vi "Untitled 1.vi"() -> ()   [LabVIEW 2018]
uses:
  C:/Users/bowenm/Git/Acquisition/Instruments/ImagingPyrometer/Kineses/Thorlabs.MotionControl.Controls.dll
  Kineses/Thorlabs.MotionControl.Controls.dll
  C:/Users/bowenm/Git/Acquisition/Instruments/ImagingPyrometer/Kineses/ThorLabs.MotionControl.KCube.DCServoCLI.dll
  Kineses/ThorLabs.MotionControl.KCube.DCServoCLI.dll
  Global Variables.vi
  <vilib>/Utility/file.llb/Read Delimited Spreadsheet (string).vi
  <instrlib>/Thorlabs_FW102C/Thorlabs_FW102C.lvlib
panel:
  in  "Stop":bool
  out "NDFW102C out 2":i32
  out "tdms file out 2":refnum<k34>
  out "RFW102C out 2":i32=1
  out "TFW102C out 2":i32
  out "MotorMoving 2":bool
  out "Device 2":refnum<k24>
  in  "KCubeDCServoControl 2":refnum<k24>(container)
  out "NDFW102C out":i32
  in  "NDFW Serial Port":string="COM5"
  out "tdms file out":refnum<k34>
  out "RFW wls":string[](array[string])=["1000", "850", "800", "700", "650", "600"]
  out "TFW wls":string[](array[string])=["900", "850", "800", "750", "700", "600"]
  in  "Tab Control":enum32{"400-700nm", "700-1100nm"}(tab)
  in  "VisTFW Wavelength":u16(ring) caption="Wavelength 1" items=["600", "700"]
  in  "VisRFW Wavelength":u16(ring) caption="Wavelength 2" items=["600", "650", "700"]
  in  "NIRRFW Wavelengths":u16(ring) caption="Wavelength 2" items=["700", "800", "850", "1000"]
  in  "NIRTFW Wavelengths":u16(ring) caption="Wavelength 1" items=["700", "750", "800", "850", "900"]
  out "NDFs":dbl[](array[numeric])=[0.0, 0.2, 0.4, 0.5, 0.6, 1.0]
  in  "NeutralDensityFilter":u16(ring) items=["0", "0.2", "0.4", "0.5", "0.6", "1"]
  out "RFW102C out":i32=1
  in  "RFW Serial Port":string="COM3"
  out "error out":errorcluster
  out "TFW102C out":i32
  in  "TFW Serial Port":string="COM4"
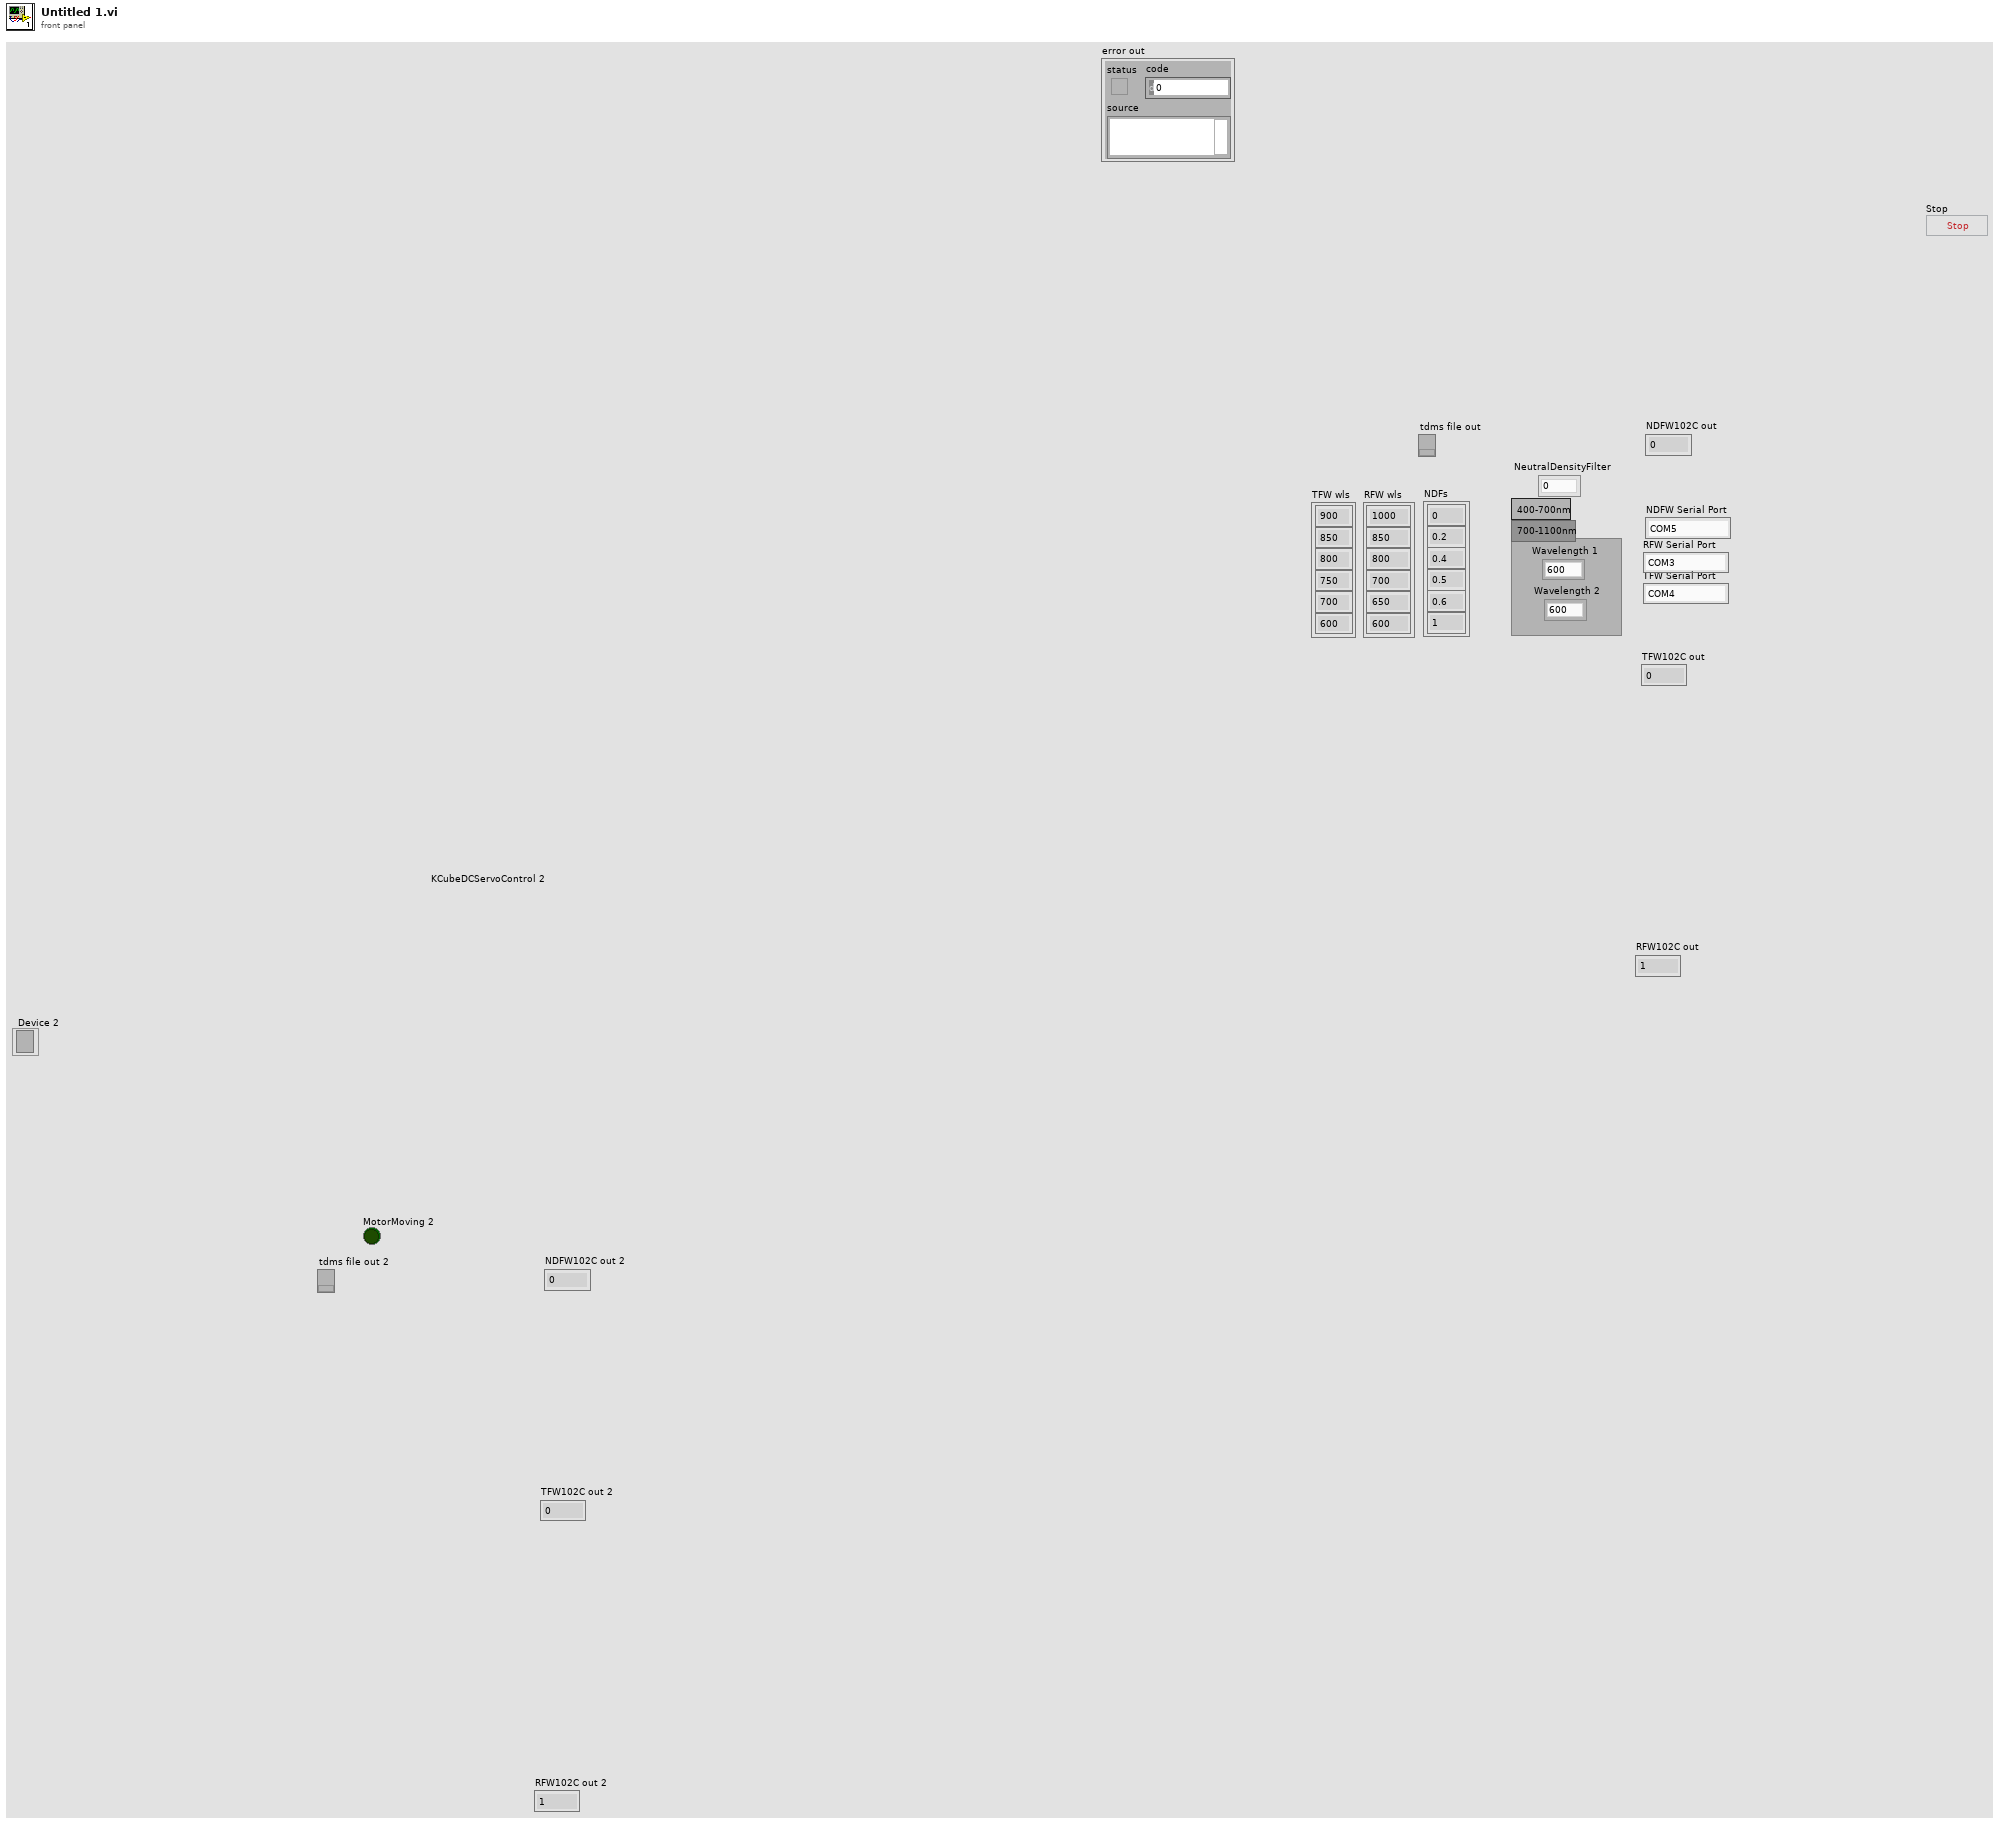
[diagram p1: front panel]
types:
  T1 = enum16{"open", "open or create", "create or replace", "create", "open (read-only)"}
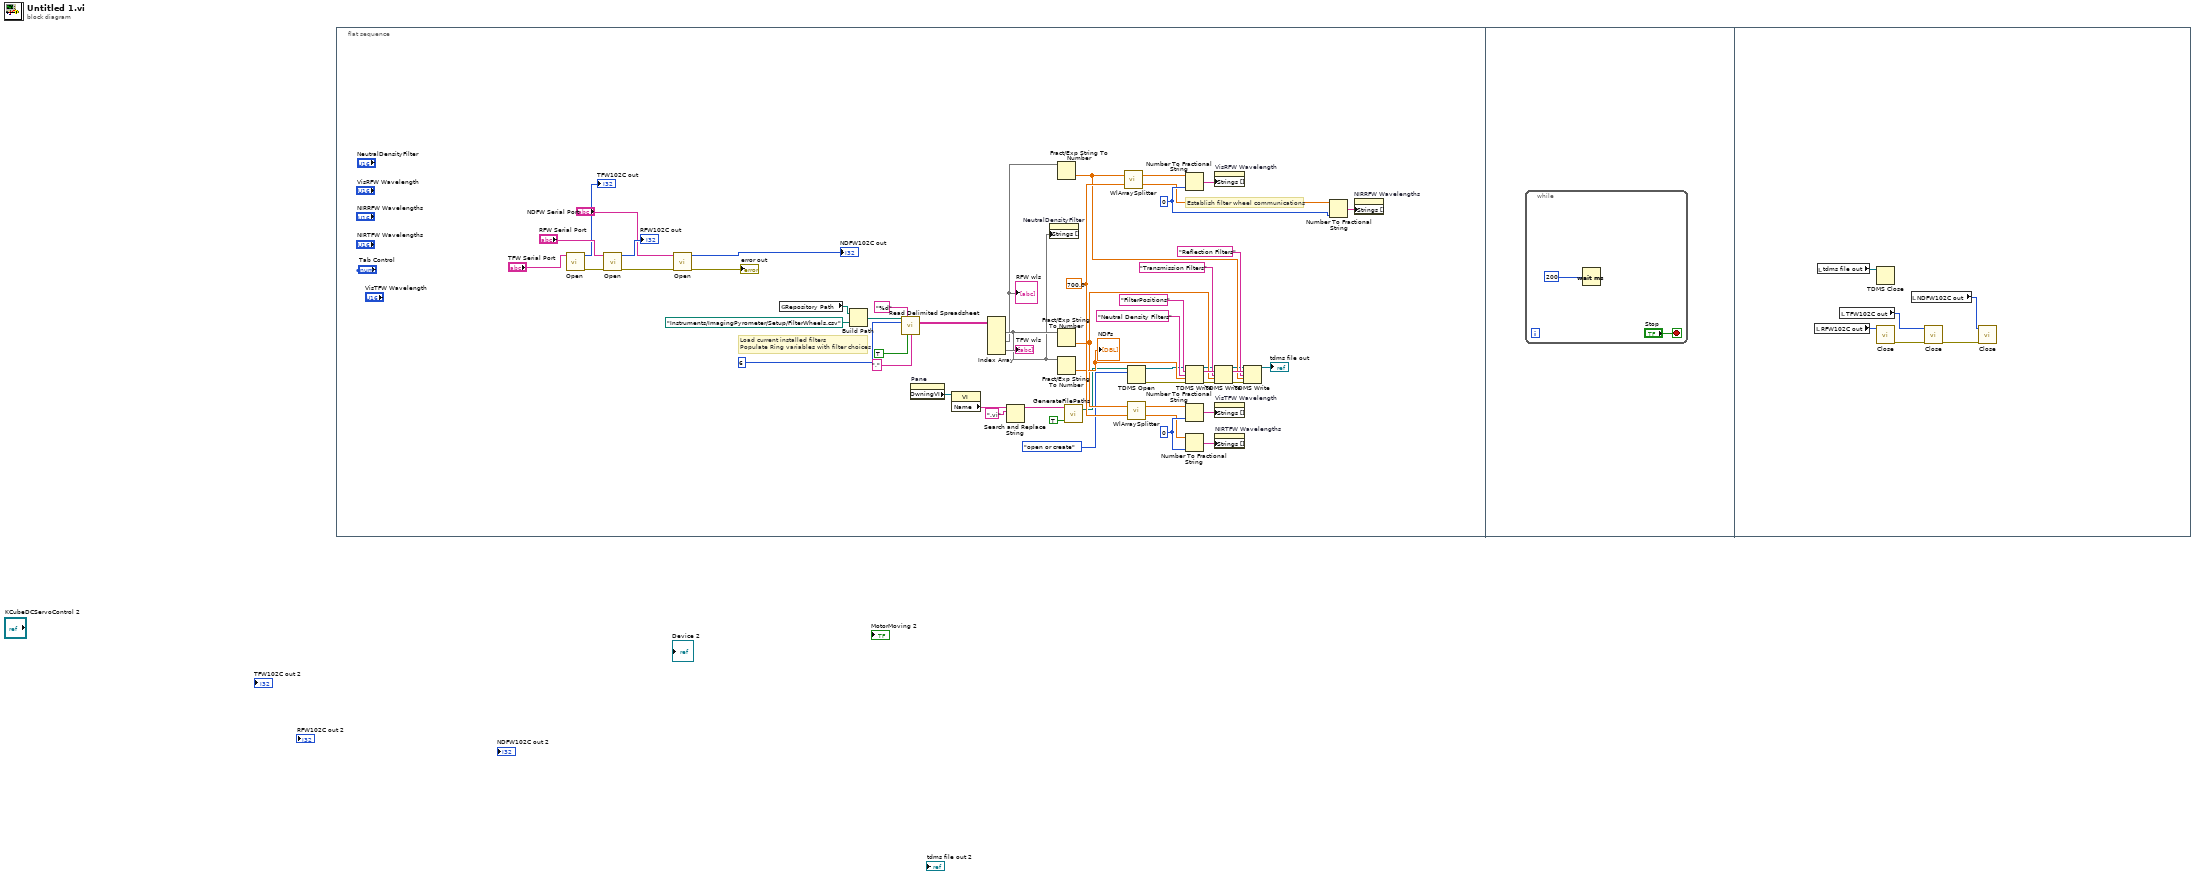
[diagram p0: block diagram]
diagram:
  n1 = flat-sequence {
    frame #0 {
      w31 = i16 0 ("precision (6)")
      w32 = 700.0 ("Cutoff Wavelength")
      w41 = i16 0 ("precision (6)")
      # "Load current installed filters\nPopulate Ring variables with filter choices"
      # "Establish filter wheel communications"
      n2 = call <instrlib>:"Open.vi"("Serial Port"="TFW Serial Port") -> ("error out"=w52:errorcluster, "FW102C out"=→"TFW102C out":i32)  [unwired: 8 in, 1 out]
      n3 = call <instrlib>:"Open.vi"("error in (no error)"=w52, "Serial Port"="RFW Serial Port") -> ("error out"=w53:errorcluster, "FW102C out"=→"RFW102C out":i32)  [unwired: 7 in, 1 out]
      n4 = call <instrlib>:"Open.vi"("error in (no error)"=w53, "Serial Port"="NDFW Serial Port") -> ("error out"=→"error out":errorcluster, "FW102C out"=→"NDFW102C out":i32)  [unwired: 7 in, 1 out]
      n5 = global read "Global Variables.vi" "Repository Path"() -> (w43:path)
      n6 = Build Path(base path=w43, name or relative path=path "Instruments/ImagingPyrometer/Setup/FilterWheels.csv" ("vi path")) -> (appended path=w44:path)
      n7 = call-poly <vilib>:"Read Delimited Spreadsheet.vi"("file path (dialog if empty)"=w44, "format (%s)"="%d", "number of rows (all:-1)"=6, "transpose? (F)"=TRUE, "delimiter (\\t)"="," ("delimiter (\\t)")) -> ("all rows"=w36:string[][])  [unwired: 5 in, 5 out]
      n8 = property on="Pane" class="Pane"() -> ("OwningVI"=w9:refnum<vi>)  [unwired: 2 in, 2 out]
      n9 = property class="VI"(reference=w9) -> ("Name"=w5:string)  [unwired: 1 in, 2 out]
      n10 = Index Array(array=w36) -> (element #1=w34:string[], element #2=w33:string[], element #3=w26:string[])  [unwired: 6 in]
      "TFW wls" <- w34
      "RFW wls" <- w33
      n11 = Search and Replace String(input string=w5, search string=".vi") -> (result string=w7:string)  [unwired: 6 in, 3 out]
      n12 = property on="NeutralDensityFilter" class="Ring (strict)"("Strings []"=w26) -> ()  [unwired: 2 in, 2 out]
      n13 = Fract/Exp String To Number(string=w33) -> (number=w17:dbl[])  [unwired: 3 in, 1 out]
      n14 = Fract/Exp String To Number(string=w34) -> (number=w21:dbl[])  [unwired: 3 in, 1 out]
      n15 = Fract/Exp String To Number(string=w26) -> (number=w25:dbl[])  [unwired: 3 in, 1 out]
      "NDFs" <- w25
      n16 = call "GenerateFilePaths.vi"("Logfile? (F)"=TRUE ("Logfile?"), "Device Name"=w7) -> ("Path"=w4:path)  [unwired: 3 in]
      n17 = call "WlArraySplitter.vi"("Cutoff Wavelength"=w32, "Wavelength Array"=w17) -> ("Higher Wavelengths"=w29:dbl[], "Lower Wavelengths"=w30:dbl[])
      n18 = TDMS Open(10:T1."open or create" ("operation (0:open)"), 11:w4) -> (0:w15:errorcluster, 3:w16:refnum<k34>)  [unwired: 5 in]
      n19 = call "WlArraySplitter.vi"("Cutoff Wavelength"=w32, "Wavelength Array"=w21) -> ("Higher Wavelengths"=w37:dbl[], "Lower Wavelengths"=w38:dbl[])
      n20 = Number To Fractional String(number=w30, precision (6)=w31) -> (F-format string=w27:string[])  [unwired: 2 in]
      n21 = TDMS Write(0:w16, 5:"FilterPositions" ("group name in (Untitled)"), 7:"Neutral Density Filters", 9:w25, 11:w15) -> (4:w14:refnum<k34>, 6:w22:string, 15:w13:errorcluster)  [unwired: 1 in, 1 out]
      n22 = Number To Fractional String(number=w38, precision (6)=w41) -> (F-format string=w40:string[])  [unwired: 2 in]
      n23 = Number To Fractional String(number=w37, precision (6)=w41) -> (F-format string=w39:string[])  [unwired: 2 in]
      n24 = property on="VisRFW Wavelength" class="Ring (strict)"("Strings []"=w27) -> ()  [unwired: 2 in, 2 out]
      n25 = TDMS Write(0:w14, 5:w22, 7:"Transmission Filters", 9:w21, 11:w13) -> (4:w11:refnum<k34>, 6:w19:string, 15:w12:errorcluster)  [unwired: 1 in, 1 out]
      n26 = property on="VisTFW Wavelength" class="Ring (strict)"("Strings []"=w40) -> ()  [unwired: 2 in, 2 out]
      n27 = property on="NIRTFW Wavelengths" class="Ring (strict)"("Strings []"=w39) -> ()  [unwired: 2 in, 2 out]
      n28 = TDMS Write(0:w11, 5:w19, 7:"Reflection Filters", 9:w17, 11:w12) -> (4:→"tdms file out":refnum<k34>)  [unwired: 1 in, 3 out]
      n29 = Number To Fractional String(number=w29, precision (6)=w31) -> (F-format string=w28:string[])  [unwired: 2 in]
      n30 = property on="NIRRFW Wavelengths" class="Ring (strict)"("Strings []"=w28) -> ()  [unwired: 2 in, 2 out]
    }
    frame #1 {
      n31 = while {
        stop <- "Stop" stop-if-true
        n32 = Wait (ms)(milliseconds to wait=u32 200) -> ()  [unwired: 1 out]
      }
    }
    frame #2 {
      n33 = local read "RFW102C out"() -> (w59:i32)
      n34 = local read "tdms file out"() -> (w60:refnum<k34>)
      n35 = local read "TFW102C out"() -> (w58:i32)
      n36 = TDMS Close(11:w60) -> ()  [unwired: 1 in, 2 out]
      n37 = call <instrlib>:"Close.vi"("FW102C in"=w59) -> ("error out"=w57:errorcluster)  [unwired: 10 in]
      n38 = local read "NDFW102C out"() -> (w62:i32)
      n39 = call <instrlib>:"Close.vi"("error in (no error)"=w57, "FW102C in"=w58) -> ("error out"=w61:errorcluster)  [unwired: 9 in]
      n40 = call <instrlib>:"Close.vi"("error in (no error)"=w61, "FW102C in"=w62) -> ()  [unwired: 9 in, 1 out]
    }
  }
